vi "DisplacementSampleLoop.vi"   [LabVIEW 2016]
uses:
  <vilib>/rvi/DataTransferAndStorage/Container/XNode/niFpgaContainer.xnode
  <vilib>/rvi/DataTransferAndStorage/Register/Emulation/niFpgaRegisterEmulation.vi
  <vilib>/Platform/TimedLoop/XDataNode/XDataNode.xnode
  <vilib>/Platform/TimedLoop/XDataNode/nitl_modes.ctl
  <vilib>/Platform/TimedLoop/XDataNode/XDNodeRunTimeDep.lvlib
  <vilib>/Platform/TimedLoop/XDataNode/wakeup.ctl
  <vilib>/Platform/TimedLoop/XDataNode/timing_clust.ctl
  DisplacementData.ctl
  DisplacementStates.ctl
  <vilib>/rvi/FIFO/Fifo_Resource/nirvififoEmulationWrite.vi
  <vilib>/rvi/FIFO/Fifo_Resource/nirvififoEmulationRead.vi
  DisplacementErrorCodes.ctl
  <vilib>/eio/EIONode/EIONode.xnode
  <vilib>/rvi/eio/common/nirviEmuTemplateMethod_errors.vi
  DisplacementSample.ctl
  DisplacementErrorSample.ctl
types:
  T1 = typedef "DisplacementData.ctl" = cluster{"State":T2, "Sensor":u8, "Negative":bool, "Timestamp":u64, "ErrorNumber":u8, "Sample":T3, "ErrorSample":T4}
  T2 = typedef "DisplacementStates.ctl" = enum16{"WaitForTrigger", "ClearRxFIFO", "WaitForClearComplete", "WriteM", "Write0", "WriteCR", "WriteNL", "ReadFirstCharacter", "ReadDataResponse", "ReadDeliminator", "ReadSign", "ReadHundreds", "ReadTens", "ReadOnes", "ReadDecimal", "ReadTenths", "ReadHundredths", "ReadThousandths", "ReadTenThousandths", "PrepareSample", "MoveSample", "ReadErrorR", "ReadErrorDeliminator1", "ReadErrorM", "ReadError0", "ReadErrorDeliminator2", "ReadErrorNumberTens", "ReadErrorNumberOnes", "ReadErrorCR", "ParseErrorNumber", "ResponseUnknownError", "ResponseInvalidError", "ResponseTimeoutError", "SensorIndicatesInvalidCommandError", "SensorIndicatesCommunicationTimeoutError", "SensorIndicatesDataLengthError", "SensorIndicatesNumberOfParametersError", "SensorIndicatesParameterError", "SensorIndicatesCommunicationError", "SensorIndicatesIDNumberError", "SensorIndicatesExpansionLineError", "SensorIndicatesWriteControlError", "PrepareErrorCode", "MoveErrorCode"}
  T3 = typedef "DisplacementSample.ctl" = cluster{"Timestamp":u64, "TxBytes":u64, "RxBytes":u64, "TxFrames":u64, "RxFrames":u64, "Sensor1Raw":i32, "Sensor2Raw":i32, "Sensor3Raw":i32, "Sensor4Raw":i32, "Sensor5Raw":i32, "Sensor6Raw":i32, "Sensor7Raw":i32, "Sensor8Raw":i32, "Sensor1Eng":sgl, "Sensor2Eng":sgl, "Sensor3Eng":sgl, "Sensor4Eng":sgl, "Sensor5Eng":sgl, "Sensor6Eng":sgl, "Sensor7Eng":sgl, "Sensor8Eng":sgl, "PositionX":sgl, "PositionY":sgl, "PositionZ":sgl, "RotationX":sgl, "RotationY":sgl, "RotationZ":sgl}
  T4 = typedef "DisplacementErrorSample.ctl" = cluster{"Timestamp":u64, "TxBytes":u64, "RxBytes":u64, "TxFrames":u64, "RxFrames":u64, "ErrorCode":T5}
  T5 = typedef "DisplacementErrorCodes.ctl" = enum16{"None", "ResponseUnknownError", "ResponseInvalidError", "ResponseTimeoutError", "SensorIndicatesInvalidCommandError", "SensorIndicatesCommunicationTimeoutError", "SensorIndicatesDataLengthError", "SensorIndicatesNumberOfParametersError", "SensorIndicatesParameterError", "SensorIndicatesCommunicationError", "SensorIndicatesIDNumberError", "SensorIndicatesExpansionLineError", "SensorIndicatesWriteControlError"}
  T6 = typedef "XDNodeRunTimeDep.lvlib/timing_clust.ctl" = cluster{"Expected End [f-1]":u64, "Actual End [f-1]":u64, "Finished Late? [f-1]":bool, "Expected End [i-1]":u64, "Actual End [i-1]":u64, "Finished Late? [i-1]":bool, "Expected Start [i]":u64, "Actual Start [i]":u64, "Expected Start [f]":u64, "Actual Start [f]":u64, "Source Name":string, "Structure Name":string, "Period":i64, "Deadline":i64, "Offset":i64, "Start":i64, "Priority":i32, "Timeout":i32, "Mode":T7, "Wakeup Reason":T8, "Error":errorcluster, "Source Type":string, "Secondary Source Type":string, "Global End Time":u64, "Global Start Time":u64, "Frame Duration":u64, "Iteration Duration":u64, "Assigned CPU":i32, "I/O Scan Engine Mode":u32}
  T7 = typedef "XDNodeRunTimeDep.lvlib/nitl_modes.ctl" = enum32{"No Change", "Process missed periods, maintain original phase", "Discard missed periods, maintain original phase", "Process missed periods, ignore original phase", "Discard missed periods, ignore original phase"}
  T8 = typedef "XDNodeRunTimeDep.lvlib/wakeup.ctl" = enum32{"Normal", "Aborted", "Asynchronous wakeup", "Timing source error", "Timed loop error", "Timeout"}
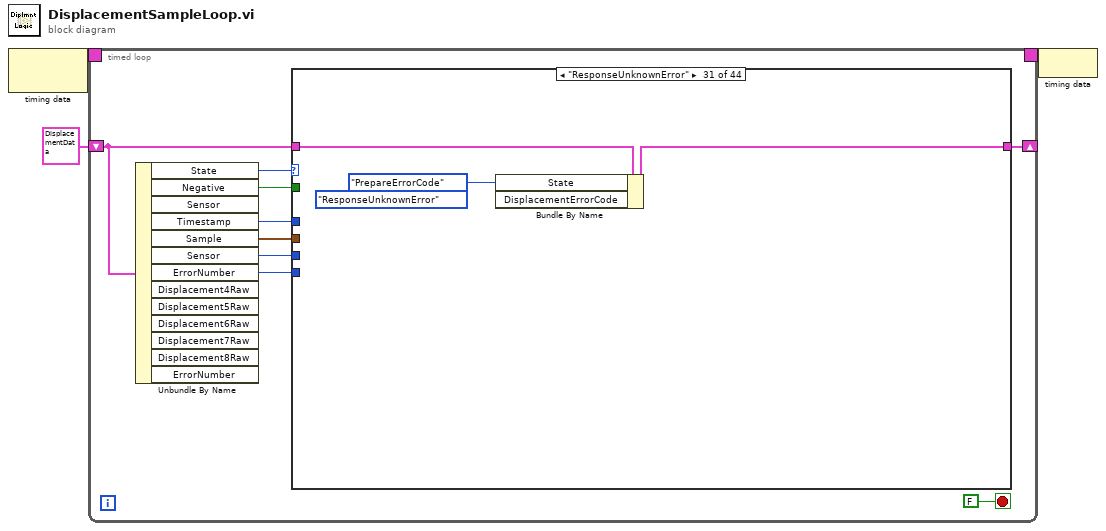
[diagram p0: block diagram]
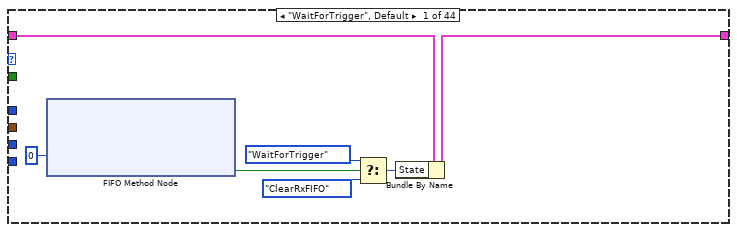
[diagram p2: hidden frame]
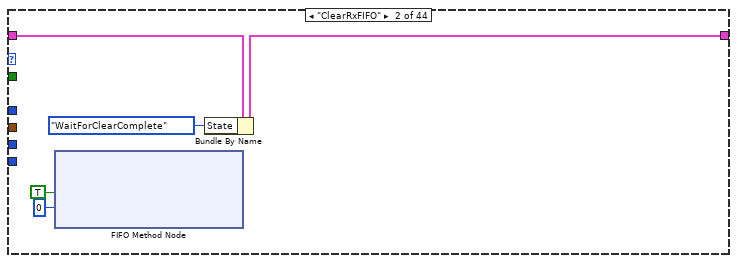
[diagram p3: hidden frame]
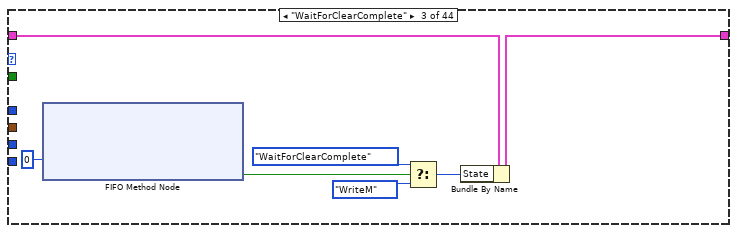
[diagram p4: hidden frame]
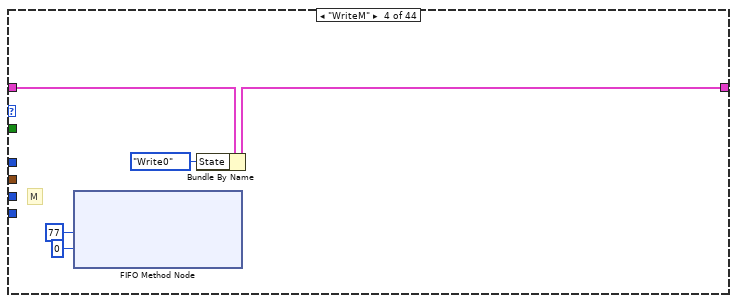
[diagram p5: hidden frame]
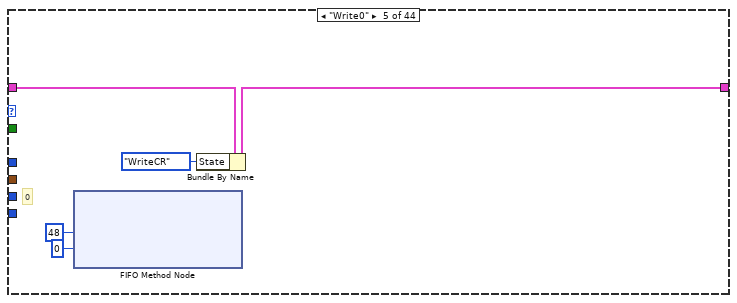
[diagram p6: hidden frame]
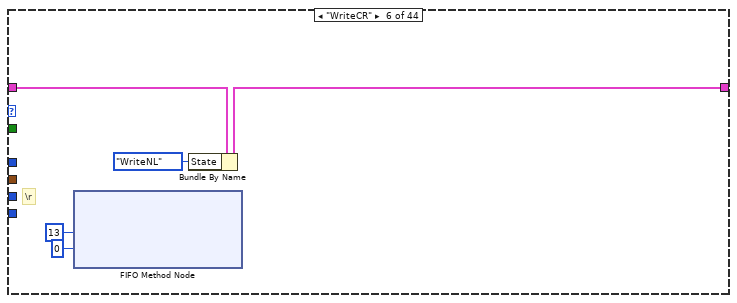
[diagram p7: hidden frame]
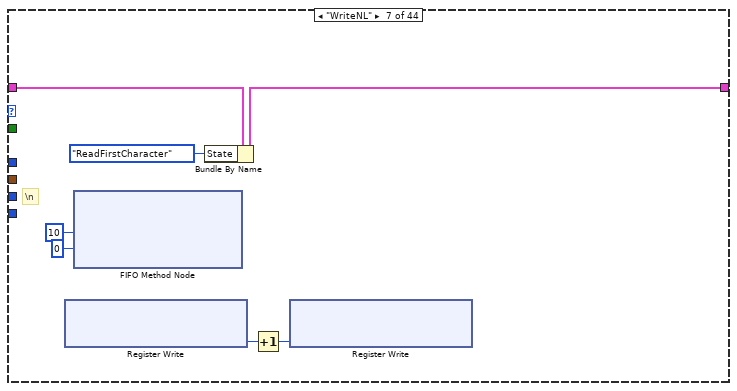
[diagram p8: hidden frame]
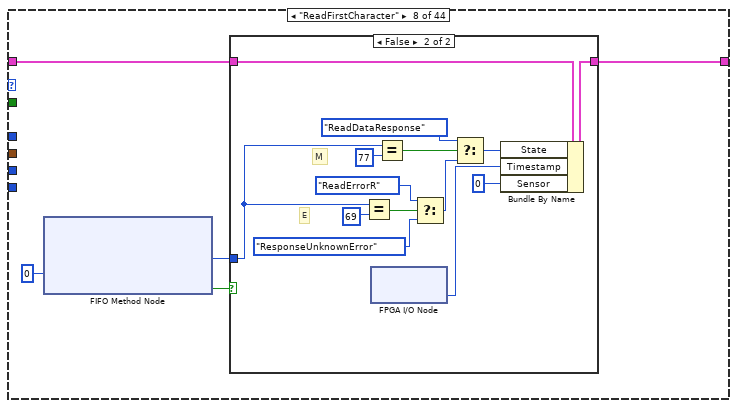
[diagram p9: hidden frame]
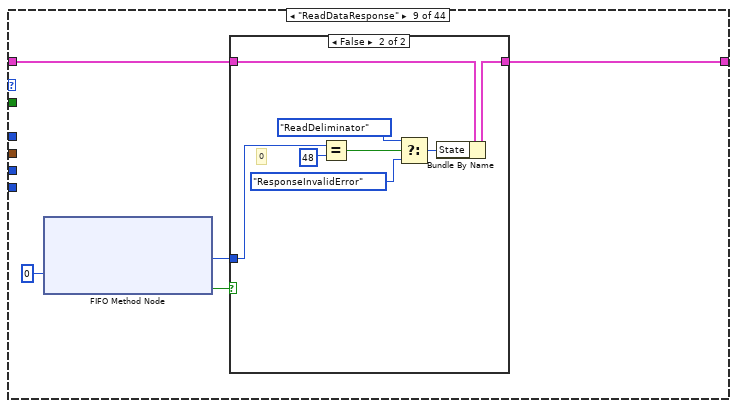
[diagram p11: hidden frame]
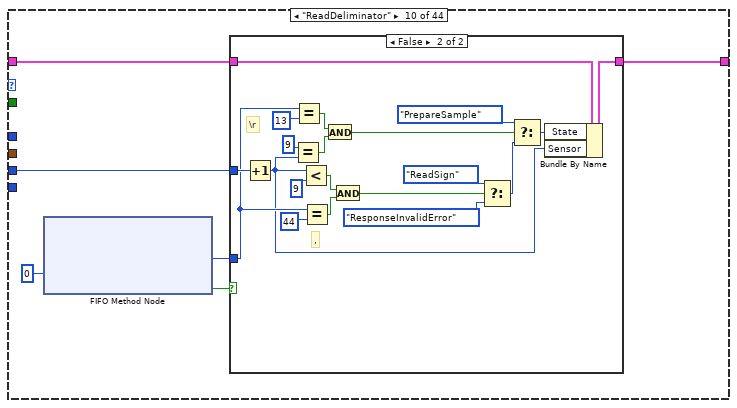
[diagram p13: hidden frame]
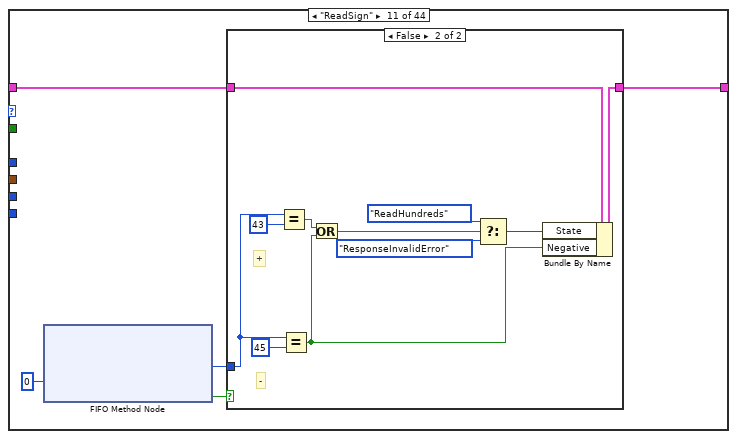
[diagram p15: hidden frame]
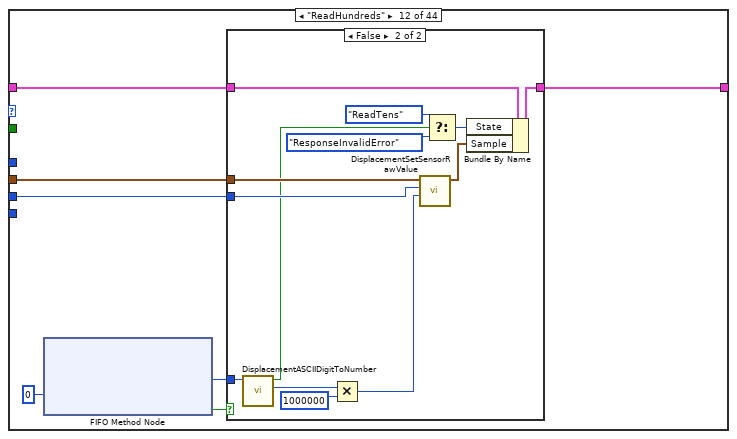
[diagram p17: hidden frame]
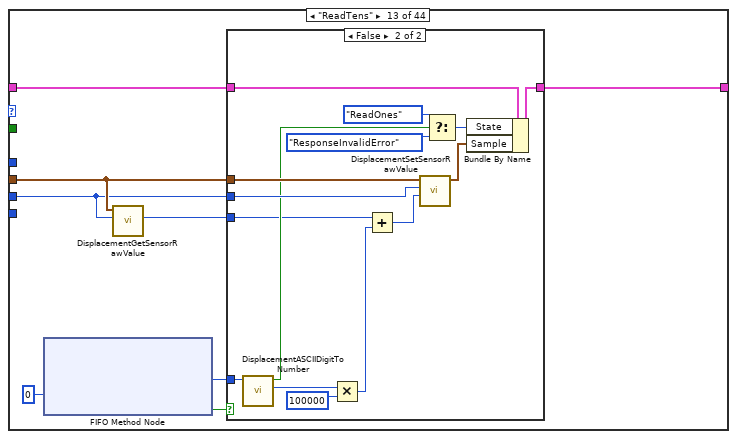
[diagram p19: hidden frame]
diagram:
  n1 = node-c288() -> (w3:T6)  [unwired: 1 in]
  n2 = timed-loop {
    timing: w3 -> [_]
    timing-out: [_] -> w2
    shift-right: [w12] -> _
    shift-left: T1 {"State"=enum."WaitForTrigger", "Sensor"=0, "Negative"=FALSE, "Timestamp"=0, "ErrorNumber"=0, "Sample"={"Timestamp"=0, "TxBytes"=0, "RxBytes"=0, "TxFrames"=0, "RxFrames"=0, "Sensor1Raw"=0, "Sensor2Raw"=0, "Sensor3Raw"=0, "Sensor4Raw"=0, "Sensor5Raw"=0, "Sensor6Raw"=0, "Sensor7Raw"=0, "Sensor8Raw"=0, "Sensor1Eng"=0.0, "Sensor2Eng"=0.0, "Sensor3Eng"=0.0, "Sensor4Eng"=0.0, "Sensor5Eng"=0.0, "Sensor6Eng"=0.0, "Sensor7Eng"=0.0, "Sensor8Eng"=0.0, "PositionX"=0.0, "PositionY"=0.0, "PositionZ"=0.0, "RotationX"=0.0, "RotationY"=0.0, "RotationZ"=0.0}, "ErrorSample"={"Timestamp"=0, "TxBytes"=0, "RxBytes"=0, "TxFrames"=0, "RxFrames"=0, "ErrorCode"=enum."None"}} ("DisplacementData") -> [w11]
    stop <- FALSE stop-if-true
    n3 = Unbundle By Name(w11) -> ("State"=w10:T2, "Negative"=w8:bool, "Timestamp"=w6:u64, "Sample"=w7:T3, "Sensor"=w5:u8, "ErrorNumber"=w4:u8)  [unwired: 7 out]
    n4 = case shown="\"ResponseUnknownError\"" w10 {
      tunnel: [w16 w23 w30 w35 w40 w45 w52 w57 w77 w92 w118 w137 w159 w183 w204 w221 w245 w269 w293 w319 w326 w330 w344 w358 w372 w386 w400 w418 w435 w447 w460 w463 w466 w469 w472 w475 w478 w481 w484 w487 w490 w493 w498 w504] -> w12
      tunnel: w11 -> [w19 w24 w31 w36 w41 w46 w53 w58 w78 w93 w119 w138 w160 w184 w205 w222 w246 w270 w294 w320 w323 w331 w345 w359 w373 w387 w401 w419 w436 w448 w461 w464 w467 w470 w473 w476 w479 w482 w485 w488 w491 w494 w499 w501]
      tunnel: w8 -> [_ _ _ _ _ _ _ _ _ _ _ _ _ _ _ _ _ _ _ _ _ _ _ _ _ _ _ _ _ _ _ _ _ _ _ _ _ _ _ _ _ _ _ _]
      tunnel: w7 -> [_ _ _ _ _ _ _ _ _ _ _ w133 w155 w179 _ w217 w241 w265 w289 _ _ _ _ _ _ _ _ _ _ _ _ _ _ _ _ _ _ _ _ _ _ _ _ _]
      tunnel: w6 -> [_ _ _ _ _ _ _ _ _ _ _ _ _ _ _ _ _ _ _ w311 _ _ _ _ _ _ _ _ _ _ _ _ _ _ _ _ _ _ _ _ _ _ _ _]
      tunnel: w5 -> [_ _ _ _ _ _ _ _ _ w88 _ w132 w154 w178 _ w216 w240 w264 w288 _ _ _ _ _ _ _ _ _ _ _ _ _ _ _ _ _ _ _ _ _ _ _ _ _]
      tunnel: w4 -> [_ _ _ _ _ _ _ _ _ _ _ _ _ _ _ _ _ _ _ _ _ _ _ _ _ _ _ w414 _ _ _ _ _ _ _ _ _ _ _ _ _ _ _ _]
      frame "WaitForTrigger", Default {
        n5 = xnode ("FIFO Method Node")("Timeout"=0) -> ("Timed Out?"=w14:bool)  [unwired: 1 in, 2 out]
        n6 = Select(t=DisplacementStates."WaitForTrigger" ("DisplacementStates"), s=w14, f=DisplacementStates."ClearRxFIFO") -> (s? t:f=w17:T2)
        n7 = Bundle By Name(cluster=w19, "State"=w17) -> (w16:T1)
      }
      frame "ClearRxFIFO" {
        n8 = xnode ("FIFO Method Node")("Element"=TRUE, "Timeout"=0) -> ()  [unwired: 1 in, 2 out]
        n9 = Bundle By Name(cluster=w24, "State"=DisplacementStates."WaitForClearComplete") -> (w23:T1)
      }
      frame "WaitForClearComplete" {
        n10 = xnode ("FIFO Method Node")("Timeout"=0) -> ("Timed Out?"=w26:bool)  [unwired: 1 in, 2 out]
        n11 = Select(t=DisplacementStates."WaitForClearComplete" ("State"), s=w26, f=DisplacementStates."WriteM") -> (s? t:f=w28:T2)
        n12 = Bundle By Name(cluster=w31, "State"=w28) -> (w30:T1)
      }
      frame "WriteM" {
        # "M"
        n13 = xnode ("FIFO Method Node")("Element"=u8 77, "Timeout"=0) -> ()  [unwired: 1 in, 2 out]
        n14 = Bundle By Name(cluster=w36, "State"=DisplacementStates."Write0" ("f")) -> (w35:T1)
      }
      frame "Write0" {
        # "0"
        n15 = xnode ("FIFO Method Node")("Element"=u8 48, "Timeout"=0) -> ()  [unwired: 1 in, 2 out]
        n16 = Bundle By Name(cluster=w41, "State"=DisplacementStates."WriteCR" ("f")) -> (w40:T1)
      }
      frame "WriteCR" {
        # "\\r"
        n17 = xnode ("FIFO Method Node")("Element"=u8 13, "Timeout"=0) -> ()  [unwired: 1 in, 2 out]
        n18 = Bundle By Name(cluster=w46, "State"=DisplacementStates."WriteNL" ("f")) -> (w45:T1)
      }
      frame "WriteNL" {
        # "\\n"
        n19 = xnode "Register Write"() -> ("Data"=w47:u64)  [unwired: 1 in, 1 out]
        n20 = xnode ("FIFO Method Node")("Element"=u8 10, "Timeout"=0) -> ()  [unwired: 1 in, 2 out]
        n21 = Bundle By Name(cluster=w53, "State"=DisplacementStates."ReadFirstCharacter") -> (w52:T1)
        n22 = Increment(x=w47) -> (x+1=w48:u64)
        n23 = xnode "Register Write"("Data"=w48) -> ()  [unwired: 1 in, 1 out]
      }
      frame "ReadFirstCharacter" {
        n24 = xnode ("FIFO Method Node")("Timeout"=0) -> ("Element"=w54:u8, "Timed Out?"=w55:bool)  [unwired: 1 in, 1 out]
        n25 = case shown="False" w55 {
          tunnel: w58 -> [w59 w73]
          tunnel: [w59 w72] -> w57
          tunnel: w54 -> [_ w65]
          frame True {
          }
          frame False {
            # "E"
            # "M"
            n26 = Equal?(x=w65, y=u8 69) -> (x = y?=w66:bool)
            n27 = xnode "FPGA I/O Node"() -> ("Time"=w61:u64)  [unwired: 1 in, 1 out]
            n28 = Equal?(x=w65, y=u8 77) -> (x = y?=w70:bool)
            n29 = Select(t=DisplacementStates."ReadErrorR", s=w66, f=DisplacementStates."ResponseUnknownError") -> (s? t:f=w63:T2)
            n30 = Select(t=DisplacementStates."ReadDataResponse" ("State"), s=w70, f=w63) -> (s? t:f=w69:T2)
            n31 = Bundle By Name(cluster=w73, "State"=w69, "Timestamp"=w61, "Sensor"=u8 0) -> (w72:T1)
          }
        }
      }
      frame "ReadDataResponse" {
        n32 = xnode ("FIFO Method Node")("Timeout"=0) -> ("Element"=w74:u8, "Timed Out?"=w75:bool)  [unwired: 1 in, 1 out]
        n33 = case shown="False" w75 {
          tunnel: w78 -> [w79 w87]
          tunnel: [w79 w86] -> w77
          tunnel: w74 -> [_ w81]
          frame True {
          }
          frame False {
            # "0"
            n34 = Equal?(x=w81, y=u8 48) -> (x = y?=w84:bool)
            n35 = Select(t=DisplacementStates."ReadDeliminator" ("State"), s=w84, f=DisplacementStates."ResponseInvalidError") -> (s? t:f=w83:T2)
            n36 = Bundle By Name(cluster=w87, "State"=w83) -> (w86:T1)
          }
        }
      }
      frame "ReadDeliminator" {
        n37 = xnode ("FIFO Method Node")("Timeout"=0) -> ("Element"=w89:u8, "Timed Out?"=w90:bool)  [unwired: 1 in, 1 out]
        n38 = case shown="False" w90 {
          tunnel: w93 -> [w94 w114]
          tunnel: [w94 w113] -> w92
          tunnel: w89 -> [_ w103]
          tunnel: w88 -> [_ w110]
          frame True {
          }
          frame False {
            # "\\r"
            # ","
            n39 = Increment(x=w110) -> (x+1=w95:u8)
            n40 = Equal?(x=u8 9, y=w95) -> (x = y?=w102:bool)
            n41 = Equal?(x=w103, y=u8 13) -> (x = y?=w101:bool)
            n42 = Less?(x=w95, y=u8 9) -> (x < y?=w108:bool)
            n43 = Equal?(x=w103, y=u8 44) -> (x = y?=w107:bool)
            n44 = And(x=w101, y=w102) -> (x .and. y?=w99:bool)
            n45 = And(x=w108, y=w107) -> (x .and. y?=w96:bool)
            n46 = Select(t=DisplacementStates."ReadSign" ("State"), s=w96, f=DisplacementStates."ResponseInvalidError") -> (s? t:f=w100:T2)
            n47 = Select(t=DisplacementStates."PrepareSample", s=w99, f=w100) -> (s? t:f=w97:T2)
            n48 = Bundle By Name(cluster=w114, "State"=w97, "Sensor"=w95) -> (w113:T1)
          }
        }
      }
      frame "ReadSign" {
        n49 = xnode ("FIFO Method Node")("Timeout"=0) -> ("Element"=w115:u8, "Timed Out?"=w116:bool)  [unwired: 1 in, 1 out]
        n50 = case shown="False" w116 {
          tunnel: w119 -> [w120 w131]
          tunnel: [w120 w130] -> w118
          tunnel: w115 -> [_ w127]
          frame True {
          }
          frame False {
            # "+"
            # "-"
            n51 = Equal?(x=w127, y=u8 43) -> (x = y?=w128:bool)
            n52 = Equal?(x=w127, y=u8 45) -> (x = y?=w125:bool)
            n53 = Or(x=w128, y=w125) -> (x .or. y?=w124:bool)
            n54 = Select(t=DisplacementStates."ReadHundreds" ("State"), s=w124, f=DisplacementStates."ResponseInvalidError") -> (s? t:f=w122:T2)
            n55 = Bundle By Name(cluster=w131, "State"=w122, "Negative"=w125) -> (w130:T1)
          }
        }
      }
      frame "ReadHundreds" {
        n56 = xnode ("FIFO Method Node")("Timeout"=0) -> ("Element"=w134:u8, "Timed Out?"=w135:bool)  [unwired: 1 in, 1 out]
        n57 = case shown="False" w135 {
          tunnel: w138 -> [w139 w152]
          tunnel: [w139 w151] -> w137
          tunnel: w134 -> [_ w142]
          tunnel: w133 -> [_ w145]
          tunnel: w132 -> [_ w143]
          frame True {
          }
          frame False {
            n58 = call "DisplacementASCIIDigitToNumber.vi"("Value"=w142) -> ("Number"=w140:i32, "Valid"=w141:bool)  [unwired: 9 in]
            n59 = Multiply(x=w140, y=1000000) -> (x*y=w146:i32)
            n60 = call "DisplacementSetSensorRawValue.vi"("Value"=w146, "Sensor"=w143, "DisplacementSample in"=w145) -> ("DisplacementSample out"=w144:T3)  [unwired: 8 in]
            n61 = Select(t=DisplacementStates."ReadTens" ("State"), s=w141, f=DisplacementStates."ResponseInvalidError" ("State")) -> (s? t:f=w149:T2)
            n62 = Bundle By Name(cluster=w152, "State"=w149, "Sample"=w144) -> (w151:T1)
          }
        }
      }
      frame "ReadTens" {
        n63 = xnode ("FIFO Method Node")("Timeout"=0) -> ("Element"=w156:u8, "Timed Out?"=w157:bool)  [unwired: 1 in, 1 out]
        n64 = call "DisplacementGetSensorRawValue.vi"("Sensor"=w154, "DisplacementSample"=w155) -> ("Value"=w153:i32)  [unwired: 9 in]
        n65 = case shown="False" w157 {
          tunnel: w160 -> [w161 w176]
          tunnel: [w161 w175] -> w159
          tunnel: w156 -> [_ w167]
          tunnel: w155 -> [_ w170]
          tunnel: w154 -> [_ w168]
          tunnel: w153 -> [_ w164]
          frame True {
          }
          frame False {
            n66 = call "DisplacementASCIIDigitToNumber.vi"("Value"=w167) -> ("Number"=w165:i32, "Valid"=w166:bool)  [unwired: 9 in]
            n67 = Multiply(x=w165, y=100000) -> (x*y=w162:i32)
            n68 = Add(x=w164, y=w162) -> (x+y=w163:i32)
            n69 = call "DisplacementSetSensorRawValue.vi"("Value"=w163, "Sensor"=w168, "DisplacementSample in"=w170) -> ("DisplacementSample out"=w169:T3)  [unwired: 8 in]
            n70 = Select(t=DisplacementStates."ReadOnes" ("State"), s=w166, f=DisplacementStates."ResponseInvalidError" ("State")) -> (s? t:f=w173:T2)
            n71 = Bundle By Name(cluster=w176, "State"=w173, "Sample"=w169) -> (w175:T1)
          }
        }
      }
      frame "ReadOnes" {
        n72 = xnode ("FIFO Method Node")("Timeout"=0) -> ("Element"=w180:u8, "Timed Out?"=w181:bool)  [unwired: 1 in, 1 out]
        n73 = call "DisplacementGetSensorRawValue.vi"("Sensor"=w178, "DisplacementSample"=w179) -> ("Value"=w177:i32)  [unwired: 9 in]
        n74 = case shown="False" w181 {
          tunnel: w184 -> [w185 w200]
          tunnel: [w185 w199] -> w183
          tunnel: w180 -> [_ w191]
          tunnel: w179 -> [_ w194]
          tunnel: w178 -> [_ w192]
          tunnel: w177 -> [_ w188]
          frame True {
          }
          frame False {
            n75 = call "DisplacementASCIIDigitToNumber.vi"("Value"=w191) -> ("Number"=w189:i32, "Valid"=w190:bool)  [unwired: 9 in]
            n76 = Multiply(x=w189, y=10000) -> (x*y=w186:i32)
            n77 = Add(x=w188, y=w186) -> (x+y=w187:i32)
            n78 = call "DisplacementSetSensorRawValue.vi"("Value"=w187, "Sensor"=w192, "DisplacementSample in"=w194) -> ("DisplacementSample out"=w193:T3)  [unwired: 8 in]
            n79 = Select(t=DisplacementStates."ReadDecimal" ("State"), s=w190, f=DisplacementStates."ResponseInvalidError" ("State")) -> (s? t:f=w197:T2)
            n80 = Bundle By Name(cluster=w200, "State"=w197, "Sample"=w193) -> (w199:T1)
          }
        }
      }
      frame "ReadDecimal" {
        n81 = xnode ("FIFO Method Node")("Timeout"=0) -> ("Element"=w201:u8, "Timed Out?"=w202:bool)  [unwired: 1 in, 1 out]
        n82 = case shown="False" w202 {
          tunnel: w205 -> [w206 w214]
          tunnel: [w206 w213] -> w204
          tunnel: w201 -> [_ w209]
          frame True {
          }
          frame False {
            # "."
            n83 = Equal?(x=w209, y=u8 46) -> (x = y?=w207:bool)
            n84 = Select(t=DisplacementStates."ReadTenths" ("State"), s=w207, f=DisplacementStates."ResponseInvalidError" ("State")) -> (s? t:f=w212:T2)
            n85 = Bundle By Name(cluster=w214, "State"=w212) -> (w213:T1)
          }
        }
      }
      frame "ReadTenths" {
        n86 = xnode ("FIFO Method Node")("Timeout"=0) -> ("Element"=w218:u8, "Timed Out?"=w219:bool)  [unwired: 1 in, 1 out]
        n87 = call "DisplacementGetSensorRawValue.vi"("Sensor"=w216, "DisplacementSample"=w217) -> ("Value"=w215:i32)  [unwired: 9 in]
        n88 = case shown="False" w219 {
          tunnel: w222 -> [w223 w238]
          tunnel: [w223 w237] -> w221
          tunnel: w218 -> [_ w229]
          tunnel: w217 -> [_ w232]
          tunnel: w216 -> [_ w230]
          tunnel: w215 -> [_ w226]
          frame True {
          }
          frame False {
            n89 = call "DisplacementASCIIDigitToNumber.vi"("Value"=w229) -> ("Number"=w227:i32, "Valid"=w228:bool)  [unwired: 9 in]
            n90 = Multiply(x=w227, y=1000) -> (x*y=w224:i32)
            n91 = Add(x=w226, y=w224) -> (x+y=w225:i32)
            n92 = call "DisplacementSetSensorRawValue.vi"("Value"=w225, "Sensor"=w230, "DisplacementSample in"=w232) -> ("DisplacementSample out"=w231:T3)  [unwired: 8 in]
            n93 = Select(t=DisplacementStates."ReadHundredths" ("State"), s=w228, f=DisplacementStates."ResponseInvalidError" ("State")) -> (s? t:f=w235:T2)
            n94 = Bundle By Name(cluster=w238, "State"=w235, "Sample"=w231) -> (w237:T1)
          }
        }
      }
      frame "ReadHundredths" {
        n95 = xnode ("FIFO Method Node")("Timeout"=0) -> ("Element"=w242:u8, "Timed Out?"=w243:bool)  [unwired: 1 in, 1 out]
        n96 = call "DisplacementGetSensorRawValue.vi"("Sensor"=w240, "DisplacementSample"=w241) -> ("Value"=w239:i32)  [unwired: 9 in]
        n97 = case shown="False" w243 {
          tunnel: w246 -> [w247 w262]
          tunnel: [w247 w261] -> w245
          tunnel: w242 -> [_ w253]
          tunnel: w241 -> [_ w256]
          tunnel: w240 -> [_ w254]
          tunnel: w239 -> [_ w250]
          frame True {
          }
          frame False {
            n98 = call "DisplacementASCIIDigitToNumber.vi"("Value"=w253) -> ("Number"=w251:i32, "Valid"=w252:bool)  [unwired: 9 in]
            n99 = Multiply(x=w251, y=100) -> (x*y=w248:i32)
            n100 = Add(x=w250, y=w248) -> (x+y=w249:i32)
            n101 = call "DisplacementSetSensorRawValue.vi"("Value"=w249, "Sensor"=w254, "DisplacementSample in"=w256) -> ("DisplacementSample out"=w255:T3)  [unwired: 8 in]
            n102 = Select(t=DisplacementStates."ReadThousandths" ("State"), s=w252, f=DisplacementStates."ResponseInvalidError" ("State")) -> (s? t:f=w259:T2)
            n103 = Bundle By Name(cluster=w262, "State"=w259, "Sample"=w255) -> (w261:T1)
          }
        }
      }
      frame "ReadThousandths" {
        n104 = xnode ("FIFO Method Node")("Timeout"=0) -> ("Element"=w266:u8, "Timed Out?"=w267:bool)  [unwired: 1 in, 1 out]
        n105 = call "DisplacementGetSensorRawValue.vi"("Sensor"=w264, "DisplacementSample"=w265) -> ("Value"=w263:i32)  [unwired: 9 in]
        n106 = case shown="False" w267 {
          tunnel: w270 -> [w271 w286]
          tunnel: [w271 w285] -> w269
          tunnel: w266 -> [_ w277]
          tunnel: w265 -> [_ w280]
          tunnel: w264 -> [_ w278]
          tunnel: w263 -> [_ w274]
          frame True {
          }
          frame False {
            n107 = call "DisplacementASCIIDigitToNumber.vi"("Value"=w277) -> ("Number"=w275:i32, "Valid"=w276:bool)  [unwired: 9 in]
            n108 = Multiply(x=w275, y=10) -> (x*y=w272:i32)
            n109 = Add(x=w274, y=w272) -> (x+y=w273:i32)
            n110 = call "DisplacementSetSensorRawValue.vi"("Value"=w273, "Sensor"=w278, "DisplacementSample in"=w280) -> ("DisplacementSample out"=w279:T3)  [unwired: 8 in]
            n111 = Select(t=DisplacementStates."ReadTenThousandths" ("State"), s=w276, f=DisplacementStates."ResponseInvalidError" ("State")) -> (s? t:f=w283:T2)
            n112 = Bundle By Name(cluster=w286, "State"=w283, "Sample"=w279) -> (w285:T1)
          }
        }
      }
      frame "ReadTenThousandths" {
        n113 = xnode ("FIFO Method Node")("Timeout"=0) -> ("Element"=w290:u8, "Timed Out?"=w291:bool)  [unwired: 1 in, 1 out]
        n114 = call "DisplacementGetSensorRawValue.vi"("Sensor"=w288, "DisplacementSample"=w289) -> ("Value"=w287:i32)  [unwired: 9 in]
        n115 = case shown="False" w291 {
          tunnel: w294 -> [w295 w310]
          tunnel: [w295 w309] -> w293
          tunnel: w290 -> [_ w301]
          tunnel: w289 -> [_ w304]
          tunnel: w288 -> [_ w302]
          tunnel: w287 -> [_ w298]
          frame True {
          }
          frame False {
            n116 = call "DisplacementASCIIDigitToNumber.vi"("Value"=w301) -> ("Number"=w299:i32, "Valid"=w300:bool)  [unwired: 9 in]
            n117 = Multiply(x=w299, y=1) -> (x*y=w296:i32)
            n118 = Add(x=w298, y=w296) -> (x+y=w297:i32)
            n119 = call "DisplacementSetSensorRawValue.vi"("Value"=w297, "Sensor"=w302, "DisplacementSample in"=w304) -> ("DisplacementSample out"=w303:T3)  [unwired: 8 in]
            n120 = Select(t=DisplacementStates."ReadDeliminator" ("State"), s=w300, f=DisplacementStates."ResponseInvalidError" ("State")) -> (s? t:f=w307:T2)
            n121 = Bundle By Name(cluster=w310, "State"=w307, "Sample"=w303) -> (w309:T1)
          }
        }
      }
      frame "PrepareSample" {
        n122 = xnode "Register Write"() -> ("Data"=w317:u64)  [unwired: 1 in, 1 out]
        n123 = xnode "Register Write"() -> ("Data"=w313:u64)  [unwired: 1 in, 1 out]
        n124 = xnode "Register Write"() -> ("Data"=w314:u64)  [unwired: 1 in, 1 out]
        n125 = xnode "Register Write"() -> ("Data"=w312:u64)  [unwired: 1 in, 1 out]
        n126 = Increment(x=w317) -> (x+1=w315:u64)
        n127 = xnode "Register Read"("Data"=w315) -> ()  [unwired: 1 in, 1 out]
        n128 = Bundle By Name(cluster=w320, "State"=DisplacementStates."MoveSample", "Sensor"=u8 1, "Sample.RxFrames"=w315, "Sample.TxBytes"=w314, "Sample.RxBytes"=w313, "Sample.TxFrames"=w312, "Timestamp"=w311) -> (w319:T1)
      }
      frame "MoveSample" {
        n129 = Unbundle By Name(w323) -> ("Sample"=w321:T3)
        n130 = xnode ("FIFO Method Node")("Element"=w321, "Timeout"=0) -> ()  [unwired: 1 in, 2 out]
        n131 = Bundle By Name(cluster=w323, "State"=DisplacementStates."WaitForTrigger", "Sensor"=u8 1) -> (w326:T1)
      }
      frame "ReadErrorR" {
        n132 = xnode ("FIFO Method Node")("Timeout"=0) -> ("Element"=w327:u8, "Timed Out?"=w328:bool)  [unwired: 1 in, 1 out]
        n133 = case shown="False" w328 {
          tunnel: w331 -> [w332 w340]
          tunnel: [w332 w339] -> w330
          tunnel: w327 -> [_ w334]
          frame True {
          }
          frame False {
            # "R"
            n134 = Equal?(x=w334, y=u8 82) -> (x = y?=w337:bool)
            n135 = Select(t=DisplacementStates."ReadErrorDeliminator1" ("State"), s=w337, f=DisplacementStates."ResponseInvalidError") -> (s? t:f=w336:T2)
            n136 = Bundle By Name(cluster=w340, "State"=w336) -> (w339:T1)
          }
        }
      }
      frame "ReadErrorDeliminator1" {
        n137 = xnode ("FIFO Method Node")("Timeout"=0) -> ("Element"=w341:u8, "Timed Out?"=w342:bool)  [unwired: 1 in, 1 out]
        n138 = case shown="False" w342 {
          tunnel: w345 -> [w346 w354]
          tunnel: [w346 w353] -> w344
          tunnel: w341 -> [_ w349]
          frame True {
          }
          frame False {
            # ","
            n139 = Equal?(x=w349, y=u8 44) -> (x = y?=w348:bool)
            n140 = Select(t=DisplacementStates."ReadErrorM" ("State"), s=w348, f=DisplacementStates."ResponseInvalidError") -> (s? t:f=w347:T2)
            n141 = Bundle By Name(cluster=w354, "State"=w347) -> (w353:T1)
          }
        }
      }
      frame "ReadErrorM" {
        n142 = xnode ("FIFO Method Node")("Timeout"=0) -> ("Element"=w355:u8, "Timed Out?"=w356:bool)  [unwired: 1 in, 1 out]
        n143 = case shown="False" w356 {
          tunnel: w359 -> [w360 w368]
          tunnel: [w360 w367] -> w358
          tunnel: w355 -> [_ w362]
          frame True {
          }
          frame False {
            # "M"
            n144 = Equal?(x=w362, y=u8 77) -> (x = y?=w365:bool)
            n145 = Select(t=DisplacementStates."ReadError0" ("State"), s=w365, f=DisplacementStates."ResponseInvalidError") -> (s? t:f=w364:T2)
            n146 = Bundle By Name(cluster=w368, "State"=w364) -> (w367:T1)
          }
        }
      }
      frame "ReadError0" {
        n147 = xnode ("FIFO Method Node")("Timeout"=0) -> ("Element"=w369:u8, "Timed Out?"=w370:bool)  [unwired: 1 in, 1 out]
        n148 = case shown="False" w370 {
          tunnel: w373 -> [w374 w382]
          tunnel: [w374 w381] -> w372
          tunnel: w369 -> [_ w376]
          frame True {
          }
          frame False {
            # "0"
            n149 = Equal?(x=w376, y=u8 48) -> (x = y?=w379:bool)
            n150 = Select(t=DisplacementStates."ReadErrorDeliminator2" ("State"), s=w379, f=DisplacementStates."ResponseInvalidError") -> (s? t:f=w378:T2)
            n151 = Bundle By Name(cluster=w382, "State"=w378) -> (w381:T1)
          }
        }
      }
      frame "ReadErrorDeliminator2" {
        n152 = xnode ("FIFO Method Node")("Timeout"=0) -> ("Element"=w383:u8, "Timed Out?"=w384:bool)  [unwired: 1 in, 1 out]
        n153 = case shown="False" w384 {
          tunnel: w387 -> [w388 w396]
          tunnel: [w388 w395] -> w386
          tunnel: w383 -> [_ w391]
          frame True {
          }
          frame False {
            # ","
            n154 = Equal?(x=w391, y=u8 44) -> (x = y?=w390:bool)
            n155 = Select(t=DisplacementStates."ReadErrorNumberTens" ("State"), s=w390, f=DisplacementStates."ResponseInvalidError") -> (s? t:f=w389:T2)
            n156 = Bundle By Name(cluster=w396, "State"=w389) -> (w395:T1)
          }
        }
      }
      frame "ReadErrorNumberTens" {
        n157 = xnode ("FIFO Method Node")("Timeout"=0) -> ("Element"=w397:u8, "Timed Out?"=w398:bool)  [unwired: 1 in, 1 out]
        n158 = case shown="False" w398 {
          tunnel: w401 -> [w402 w413]
          tunnel: [w402 w412] -> w400
          tunnel: w397 -> [_ w406]
          frame True {
          }
          frame False {
            n159 = call "DisplacementASCIIDigitToNumber.vi"("Value"=w406) -> ("Number"=w403:i32, "Valid"=w405:bool)  [unwired: 9 in]
            n160 = To Unsigned Byte Integer(number=w403) -> (unsigned 8bit integer=w404:u8)
            n161 = Multiply(x=w404, y=u8 10) -> (x*y=w407:u8)
            n162 = Select(t=DisplacementStates."ReadErrorNumberOnes" ("State"), s=w405, f=DisplacementStates."ResponseInvalidError" ("State")) -> (s? t:f=w410:T2)
            n163 = Bundle By Name(cluster=w413, "State"=w410, "ErrorNumber"=w407) -> (w412:T1)
          }
        }
      }
      frame "ReadErrorNumberOnes" {
        n164 = xnode ("FIFO Method Node")("Timeout"=0) -> ("Element"=w415:u8, "Timed Out?"=w416:bool)  [unwired: 1 in, 1 out]
        n165 = case shown="False" w416 {
          tunnel: w419 -> [w420 w431]
          tunnel: [w420 w430] -> w418
          tunnel: w415 -> [_ w424]
          tunnel: w414 -> [_ w425]
          frame True {
          }
          frame False {
            n166 = call "DisplacementASCIIDigitToNumber.vi"("Value"=w424) -> ("Number"=w422:i32, "Valid"=w423:bool)  [unwired: 9 in]
            n167 = To Unsigned Byte Integer(number=w422) -> (unsigned 8bit integer=w421:u8)
            n168 = Add(x=w425, y=w421) -> (x+y=w426:u8)
            n169 = Select(t=DisplacementStates."ReadErrorCR" ("State"), s=w423, f=DisplacementStates."ResponseInvalidError" ("State")) -> (s? t:f=w429:T2)
            n170 = Bundle By Name(cluster=w431, "State"=w429, "ErrorNumber"=w426) -> (w430:T1)
          }
        }
      }
      frame "ReadErrorCR" {
        n171 = xnode ("FIFO Method Node")("Timeout"=0) -> ("Element"=w432:u8, "Timed Out?"=w433:bool)  [unwired: 1 in, 1 out]
        n172 = case shown="False" w433 {
          tunnel: w436 -> [w437 w445]
          tunnel: [w437 w444] -> w435
          tunnel: w432 -> [_ w440]
          frame True {
          }
          frame False {
            # "\\r"
            n173 = Equal?(x=w440, y=u8 13) -> (x = y?=w439:bool)
            n174 = Select(t=DisplacementStates."ParseErrorNumber" ("State"), s=w439, f=DisplacementStates."ResponseInvalidError") -> (s? t:f=w438:T2)
            n175 = Bundle By Name(cluster=w445, "State"=w438) -> (w444:T1)
          }
        }
      }
      frame "ParseErrorNumber" {
        n176 = case shown="255, Default" {
          selector: _ -> [_ _ _ _ _ _ _ _ _ _]
          tunnel: [DisplacementStates."ResponseInvalidError" ("State") DisplacementStates."SensorIndicatesInvalidCommandError" ("State") DisplacementStates."SensorIndicatesCommunicationTimeoutError" ("State") DisplacementStates."SensorIndicatesDataLengthError" ("State") DisplacementStates."SensorIndicatesNumberOfParametersError" ("State") DisplacementStates."SensorIndicatesParameterError" ("State") DisplacementStates."SensorIndicatesCommunicationError" ("State") DisplacementStates."SensorIndicatesIDNumberError" ("State") DisplacementStates."SensorIndicatesExpansionLineError" ("State") DisplacementStates."SensorIndicatesWriteControlError" ("State")] -> w446
          frame 255, Default {
          }
          frame 0 {
          }
          frame 2 {
          }
          frame 20 {
          }
          frame 21 {
          }
          frame 22 {
          }
          frame 29 {
          }
          frame 65 {
          }
          frame 66 {
          }
          frame 67 {
          }
        }
        n177 = Bundle By Name(cluster=w448, "State"=w446) -> (w447:T1)
      }
      frame "ResponseUnknownError" {
        (unwired) DisplacementErrorCodes."ResponseUnknownError" ("DisplacementErrorCodes")
        n178 = Bundle By Name(cluster=w461, "State"=DisplacementStates."PrepareErrorCode") -> (w460:T1)  [unwired: 1 in]
      }
      frame "ResponseInvalidError" {
        (unwired) DisplacementErrorCodes."ResponseInvalidError" ("DisplacementErrorCodes")
        n179 = Bundle By Name(cluster=w464, "State"=DisplacementStates."PrepareErrorCode") -> (w463:T1)  [unwired: 1 in]
      }
      frame "ResponseTimeoutError" {
        (unwired) DisplacementErrorCodes."ResponseTimeoutError" ("DisplacementErrorCodes")
        n180 = Bundle By Name(cluster=w467, "State"=DisplacementStates."PrepareErrorCode") -> (w466:T1)  [unwired: 1 in]
      }
      frame "SensorIndicatesInvalidCommandError" {
        (unwired) DisplacementErrorCodes."SensorIndicatesInvalidCommandError" ("DisplacementErrorCodes")
        n181 = Bundle By Name(cluster=w470, "State"=DisplacementStates."PrepareErrorCode") -> (w469:T1)  [unwired: 1 in]
      }
      frame "SensorIndicatesCommunicationTimeoutError" {
        (unwired) DisplacementErrorCodes."SensorIndicatesCommunicationTimeoutError" ("DisplacementErrorCodes")
        n182 = Bundle By Name(cluster=w473, "State"=DisplacementStates."PrepareErrorCode") -> (w472:T1)  [unwired: 1 in]
      }
      frame "SensorIndicatesDataLengthError" {
        (unwired) DisplacementErrorCodes."SensorIndicatesDataLengthError" ("DisplacementErrorCodes")
        n183 = Bundle By Name(cluster=w476, "State"=DisplacementStates."PrepareErrorCode") -> (w475:T1)  [unwired: 1 in]
      }
      frame "SensorIndicatesNumberOfParametersError" {
        (unwired) DisplacementErrorCodes."SensorIndicatesNumberOfParametersError" ("DisplacementErrorCodes")
        n184 = Bundle By Name(cluster=w479, "State"=DisplacementStates."PrepareErrorCode") -> (w478:T1)  [unwired: 1 in]
      }
      frame "SensorIndicatesParameterError" {
        (unwired) DisplacementErrorCodes."SensorIndicatesParameterError" ("DisplacementErrorCodes")
        n185 = Bundle By Name(cluster=w482, "State"=DisplacementStates."PrepareErrorCode") -> (w481:T1)  [unwired: 1 in]
      }
      frame "SensorIndicatesCommunicationError" {
        (unwired) DisplacementErrorCodes."SensorIndicatesCommunicationError" ("DisplacementErrorCodes")
        n186 = Bundle By Name(cluster=w485, "State"=DisplacementStates."PrepareErrorCode") -> (w484:T1)  [unwired: 1 in]
      }
      frame "SensorIndicatesIDNumberError" {
        (unwired) DisplacementErrorCodes."SensorIndicatesIDNumberError" ("DisplacementErrorCodes")
        n187 = Bundle By Name(cluster=w488, "State"=DisplacementStates."PrepareErrorCode") -> (w487:T1)  [unwired: 1 in]
      }
      frame "SensorIndicatesExpansionLineError" {
        (unwired) DisplacementErrorCodes."SensorIndicatesExpansionLineError" ("DisplacementErrorCodes")
        n188 = Bundle By Name(cluster=w491, "State"=DisplacementStates."PrepareErrorCode") -> (w490:T1)  [unwired: 1 in]
      }
      frame "SensorIndicatesWriteControlError" {
        (unwired) DisplacementErrorCodes."SensorIndicatesWriteControlError" ("DisplacementErrorCodes")
        n189 = Bundle By Name(cluster=w494, "State"=DisplacementStates."PrepareErrorCode") -> (w493:T1)  [unwired: 1 in]
      }
      frame "PrepareErrorCode" {
        n190 = xnode "Register Read"() -> ("Data"=w496:u64)  [unwired: 1 in, 1 out]
        n191 = xnode "Register Read"() -> ()  [unwired: 1 in, 2 out]
        n192 = xnode "Register Read"() -> ()  [unwired: 1 in, 2 out]
        n193 = xnode "Register Read"() -> ()  [unwired: 1 in, 2 out]
        n194 = Increment(x=w496) -> ()  [unwired: 1 out]
        n195 = xnode "Register Write"() -> ()  [unwired: 2 in, 1 out]
        n196 = Bundle By Name(cluster=w499, "State"=DisplacementStates."MoveErrorCode", "Sensor"=u8 1) -> (w498:T1)  [unwired: 5 in]
      }
      frame "MoveErrorCode" {
        n197 = Unbundle By Name(w501) -> ()  [unwired: 1 out]
        n198 = xnode ("FIFO Method Node")("Timeout"=0) -> ()  [unwired: 2 in, 2 out]
        n199 = Bundle By Name(cluster=w501, "State"=DisplacementStates."WaitForTrigger", "Sensor"=u8 1) -> (w504:T1)
      }
    }
  }
  n200 = node-c288(w2) -> ()
